vi "_SetData.vi"(7 "Refs":T3, 8 "data":T1, 9 "Action in":T2 caption="Action", 10 "Display State In in":T4 caption="State", 11 "Data In in":T7) -> (1 "Action out":T2 caption="Action", 2 "Display State In out":T4 caption="State", 3 "Data In out":T7)   [LabVIEW 2017, in "UI_TimeSelector.xctl"]
uses:
  UI_TimeSelector.xctl
  Data.ctl
  State.ctl
  Typedefs/INTERNAL-DATA.ctl
  Interface/DEF-Mode.ctl
  Typedefs/INTERNAL-REFs.ctl
  <vilib>/_xctls/Action.ctl
  <vilib>/_xctls/XControlSupport.lvlib
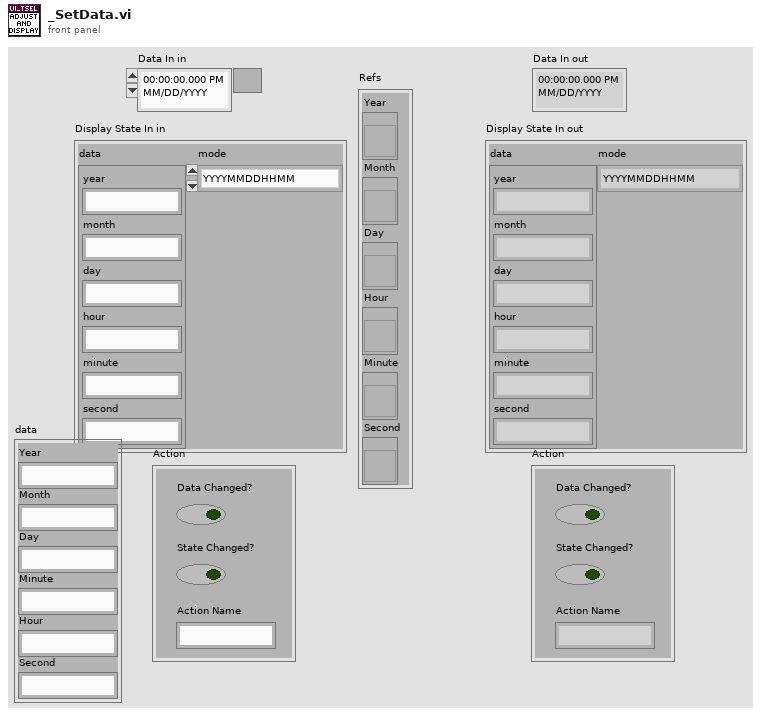
[diagram p1: front panel]
types:
  T1 = cluster{"Year":string, "Month":string, "Day":string, "Minute":string, "Hour":string, "Second":string}
  T2 = typedef "XControlSupport.lvlib/Action.ctl" = cluster{"Data Changed?":bool, "State Changed?":bool, "Action Name":string}
  T3 = typedef "UI_TimeSelector.xctl/INTERNAL-REFs.ctl" = cluster{"Year":refnum<vi>, "Month":refnum<vi>, "Day":refnum<vi>, "Hour":refnum<vi>, "Minute":refnum<vi>, "Second":refnum<vi>}
  T4 = typedef "UI_TimeSelector.xctl/State.ctl" = cluster{"data":T5, "mode":T6}
  T5 = typedef "UI_TimeSelector.xctl/INTERNAL-DATA.ctl" = cluster{"year":string, "month":string, "day":string, "hour":string, "minute":string, "second":string}
  T6 = typedef "UI_TimeSelector.xctl/DEF-Mode.ctl" = enum16{"YYYYMMDDHHMM", "YYYYMMDDHHMMSS", "YYYY", "YYYYMM", "YYYYMMDD", "HHMM", "HHMMSS"}
  T7 = typedef "UI_TimeSelector.xctl/Data.ctl" = timestamp
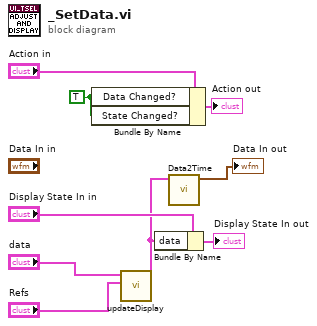
[diagram p0: block diagram]
diagram:
  w3 = TRUE ("Data Changed?")
  n1 = Bundle By Name(cluster="Action in", "Data Changed?"=w3, "State Changed?"=w3) -> (→"Action out":T2)
  n2 = call "updateDisplay.vi"("display refs"="Refs", "data"="data") -> ("data (dup)"=w1:T1)  [unwired: 9 in]
  n3 = Bundle By Name(cluster="Display State In in", "data"=w1) -> (→"Display State In out":T4)
  n4 = call "Data2Time.vi"("data"=w1) -> ("Time"=→"Data In out":timestamp)  [unwired: 10 in]
